vi "1D Quadrature Integrand for Gated Decay.vi"(10 "data":variant, 11 "X":dbl[](array[numeric])) -> (0 "Error Out":errorcluster, 3 "F(X)":dbl[](array[numeric]))   [LabVIEW 2021, in "Phasor.lvlib"]
doc: "This template is the starting point for creating a function that is the integrand evaluation to be passed to the Quadrature.vi."
uses:
  Phasor.lvlib
  Phasor Gate & Decay Parameters.ctl
  Phasor Gate Type.ctl
  Phasor IRF Model.ctl
  Graphs/XY Graph/XY Graph Plot Data.ctl
  Graphs/XY Graph/XY Graph Interpolate Plot at x.vi
  Phasor Compute Gate-IRF Array.vi/7d9bb666-8e44-4efd-bf11-38a816117c5c.vi
  Math/T-Periodic Square Gate.vi
  Math/T-Periodic Triangle Gate.vi
  Math/T-Periodic Sawtooth Gate.vi
  <vilib>/Utility/error.llb/Error Cluster From Error Code.vi
  Math/T-Periodic Finite Edge Square Gate.vi
  Math/T-Periodic Finite Edge Tilted Top Square Gate.vi
  Graphs/XY Graph/XY Graph Add-Ons.lvlib
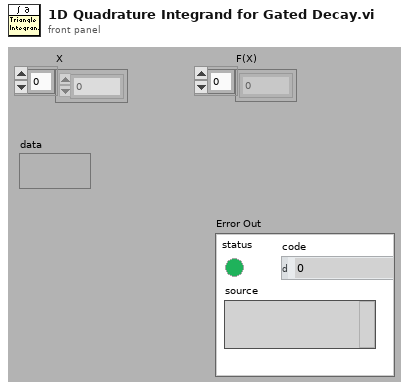
[diagram p1: front panel]
types:
  T1 = typedef "Phasor.lvlib/Phasor Gate & Decay Parameters.ctl" = cluster{"W":dbl, "T":dbl, "tau":dbl, "t_0":dbl, "Gate Type":T2, "t_i":dbl, "sR":dbl, "sF":dbl, "s":dbl, "Reversed Sawtooth":bool, "IRF Model":T3, "IRF Parameter 1":dbl, "User-defined Gate":T4, "Type of User-defined Function":enum32{"Gate", "IRF"}, "A":dbl}
  T2 = typedef "Phasor.lvlib/Phasor Gate Type.ctl" = enum16{"Square", "Finite Edge Square", "Finite Edge, Tilted Top Square", "Triangle", "Sawtooth", "User-defined"}
  T3 = typedef "Phasor.lvlib/Phasor IRF Model.ctl" = enum16{"Dirac", "Exponential"}
  T4 = typedef "XY Graph Add-Ons.lvlib/XY Graph Plot Data.ctl" = cluster{"X Array":dbl[], "Y Array":dbl[]}
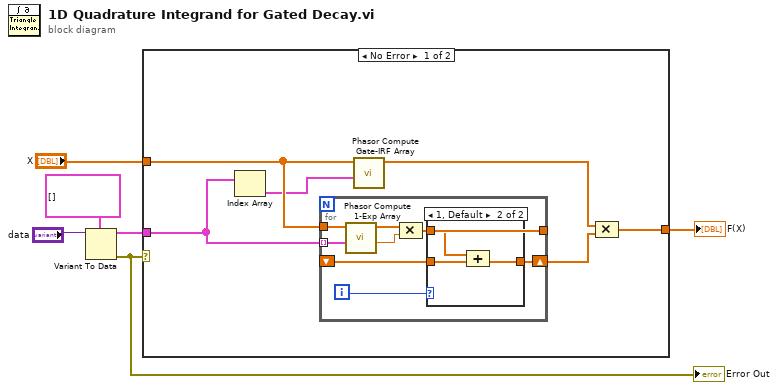
[diagram p0: block diagram]
diagram:
  n1 = Variant To Data(type=T1[] [] ("Array"), Variant="data") -> (data=w3:T1[], error out=w2:errorcluster)  [unwired: 1 in]
  "Error Out" <- w2
  n2 = case shown="No Error" w2 {
    tunnel: "X" -> [w12 _]
    tunnel: w3 -> [w10 _]
    tunnel: [w11 _] -> w1
    frame No Error {
      n3 = Index Array(array=w10) -> (element=w9:T1)  [unwired: 1 in]
      n4 = for {
        tunnel: w12 -> [w20]
        tunnel: [w14] -> _
        tunnel: w10 -> [w17] mode=indexing
        shift-right: [w15] -> w7
        shift-left: _ -> [w13]
        i -> [w16]
        n5 = call "Phasor Compute 1-Exp Array.vi"("Gate & Decay Parameters"=w17, "X"=w20) -> ("A"=w18:dbl, "1-Exp Array"=w19:dbl[])  [unwired: 7 in, 1 out]
        n6 = Compound Arithmetic op=MULTIPLY(w19, w18) -> (w14:dbl[])
        n7 = case shown="1, Default" w16 {
          tunnel: [w21 w22] -> w15
          tunnel: w14 -> [w21 w23]
          tunnel: w13 -> [_ w24]
          frame 0 {
          }
          frame 1, Default {
            n8 = Compound Arithmetic op=ADD(w23, w24) -> (w22:dbl[])
          }
        }
      }
      n9 = call "Phasor Compute Gate-IRF Array.vi"("Gate & Decay Parameters"=w9, "X"=w12) -> ("IRF/Gate Array"=w8:dbl[])  [unwired: 8 in, 1 out]
      n10 = Compound Arithmetic op=MULTIPLY(w8, w7) -> (w11:dbl[])
    }
    frame Error {
    }
  }
  "F(X)" <- w1
